vi "ControllerView.vi"() -> ()   [LabVIEW 2016]
uses:
  DataTypes/Topics/Parts/SummaryStates.ctl
  DataTypes/Topics/Parts/Timestamp.ctl
  Boot/Boot.lvclass
  UserEvents/UserEvents.lvclass/UserEvents.ctl
  DataTypes/General/ShutdownEvent.ctl
  Settings/Settings/Setting.lvclass
  UserEvents/UserEvents.lvclass
  DataTypes/General/M1M3SupportGeneral.lvlib
  DataTypes/Topics/M1M3SupportTopics.lvlib
panel:
  in  "Shutdown":bool
  out "SAL Time (ms)":i32=-123123
  in  "EditM1M3Settings":bool
  out "ModbusSubnetATxFrameCount":i32
  out "DeltaTimestamp":dbl format="%.6g"
  out "Timestamp":T1
  out "FPGATimestamp":dbl format="%.6g"
  in  "EditBaseSettings":bool
  out "SummaryStates":T2
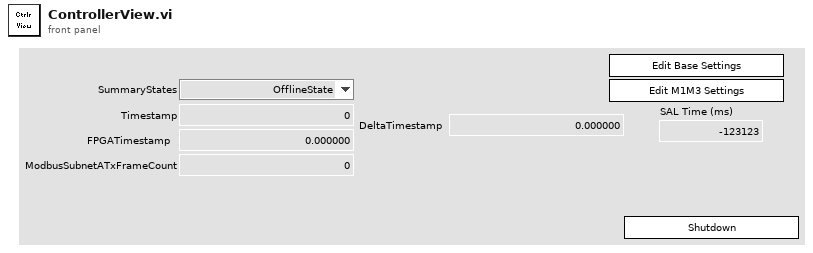
[diagram p1: front panel]
types:
  T1 = typedef "M1M3SupportTopics.lvlib/Timestamp.ctl" = dbl
  T2 = typedef "M1M3SupportTopics.lvlib/SummaryStates.ctl" = enum16{"OfflineState", "StandbyState", "DisabledState", "EnabledState", "FaultState"}
  T3 = enum32{"invalid app kind", "Development System", "Run Time System", "Student Edition", "Embedded LabVIEW", "Evaluation", "Custom"}
  T4 = typedef "M1M3SupportGeneral.lvlib/ShutdownEvent.ctl" = cluster{"Shutdown":bool}
  T5 = typedef "M1M3SupportTypes.lvlib/SummaryStates.ctl" = enum16{"OfflineState", "StandbyState", "DisabledState", "EnabledState", "FaultState"}
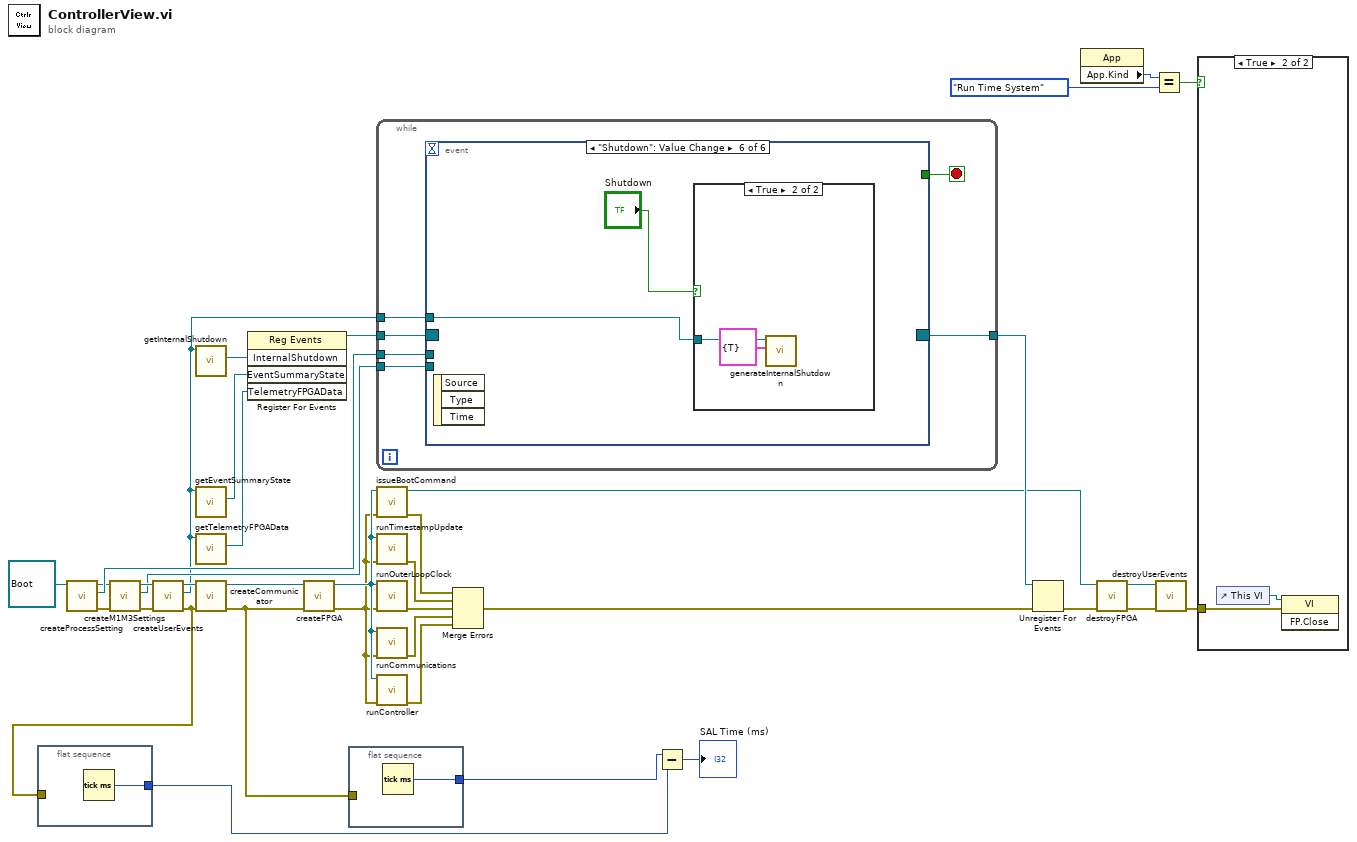
[diagram p0: block diagram]
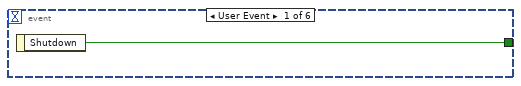
[diagram p3: hidden frame]
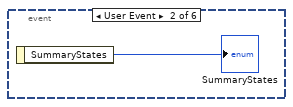
[diagram p4: hidden frame]
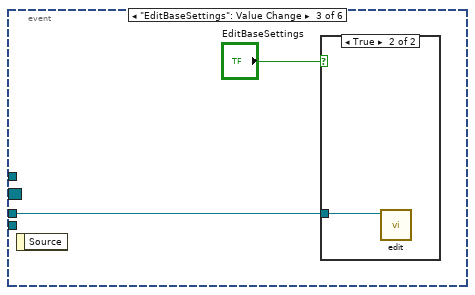
[diagram p5: hidden frame]
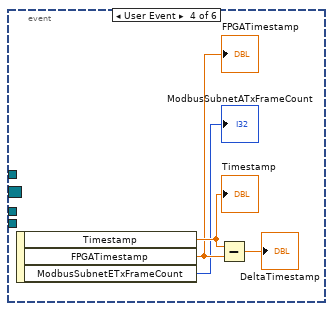
[diagram p7: hidden frame]
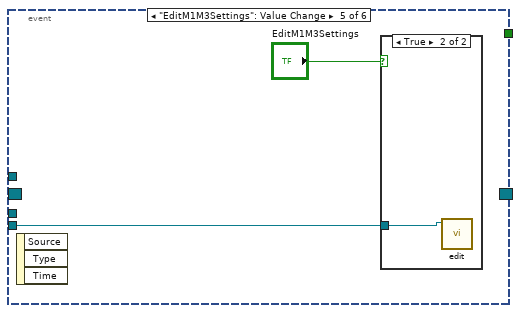
[diagram p8: hidden frame]
diagram:
  n1 = flat-sequence {
    tunnel: w6 -> [_]
    tunnel: [w37] -> w3
    frame #0 {
      n2 = Tick Count (ms)() -> (millisecond timer value=w37:u32)
    }
  }
  n3 = call "createProcessSetting.vi"("Boot in"=refnum<class "Boot.lvclass"> refnum ("Boot.lvclass")) -> ("error out"=w9:errorcluster, "ProcessSettings"=w23:refnum<class "Setting.lvclass">, "Boot out"=w11:refnum<class "Boot.lvclass">)  [unwired: 8 in]
  n4 = call "createM1M3Settings.vi"("error in (no error)"=w9, "Boot in"=w11) -> ("error out"=w8:errorcluster, "M1M3Settings"=w7:refnum<class "Setting.lvclass">, "Boot out"=w10:refnum<class "Boot.lvclass">)  [unwired: 7 in]
  n5 = call "createUserEvents.vi"("error in (no error)"=w8, "Boot in"=w10) -> ("error out"=w6:errorcluster, "UserEvents"=w1:refnum<class "UserEvents.lvclass">, "Boot out"=w14:refnum<class "Boot.lvclass">)  [unwired: 7 in]
  n6 = call "getInternalShutdown.vi"("UserEvents in"=w1) -> ("InternalShutdown"=w36:refnum<user-event>)  [unwired: 9 in, 1 out]
  n7 = call "getEventSummaryState.vi"("UserEvents in"=w1) -> ("EventSummaryState"=w35:refnum<user-event>)  [unwired: 9 in, 1 out]
  n8 = call "getTelemetryFPGAData.vi"("UserEvents in"=w1) -> ("TelemetryFPGAData"=w22:refnum<user-event>)  [unwired: 9 in, 1 out]
  n9 = call "createCommunicator.vi"("error in (no error)"=w6, "Boot in"=w14) -> ("error out"=w5:errorcluster, "Boot out"=w13:refnum<class "Boot.lvclass">)  [unwired: 7 in, 1 out]
  n10 = register-events(w36, w35, w22) -> (reference out=w34:refnum<event-registration>)  [unwired: 2 in, 1 out]
  n11 = call "createFPGA.vi"("error in (no error)"=w5, "Boot in"=w13) -> ("error out"=w20:errorcluster, "Boot out"=w21:refnum<class "Boot.lvclass">)  [unwired: 7 in, 1 out]
  n12 = flat-sequence {
    tunnel: w5 -> [_]
    tunnel: [w38] -> w4
    frame #0 {
      n13 = Tick Count (ms)() -> (millisecond timer value=w38:u32)
    }
  }
  n14 = while {
    tunnel: w34 -> [w44]
    tunnel: [w42] -> w33
    tunnel: w23 -> [w41]
    tunnel: w7 -> [w40]
    tunnel: w1 -> [w39]
    stop <- w43 stop-if-true
    n15 = event shown="[5] \"Shutdown\": Value Change" {
      selector: w44 -> [_ _ _ _ _ _]
      dyn-events: [_ _ _ _ _ _] -> w42
      timeout: _ -> [_ _ _ _ _ _]
      tunnel: [w45 _ _ _ _ _] -> w43
      tunnel: w41 -> [_ _ w47 _ _ _]
      tunnel: w40 -> [_ _ _ _ w54 _]
      tunnel: w39 -> [_ _ _ _ _ w57]
      event User Event {
        n16 = event-data() -> ("Shutdown"=w45:bool)  [unwired: 1 in]
      }
      event User Event {
        n17 = event-data() -> ("SummaryStates"=→"SummaryStates":T5)  [unwired: 1 in]
      }
      event "EditBaseSettings": Value Change {
        n18 = event-data() -> ()  [unwired: 1 in, 1 out]
        n19 = case shown="True" "EditBaseSettings" {
          tunnel: w47 -> [_ w49]
          frame False {
          }
          frame True {
            n20 = call-dynamic "edit.vi"("BaseSetting in"=w49) -> ()  [unwired: 8 in, 3 out]
          }
        }
      }
      event User Event {
        n21 = event-data() -> ("Timestamp"=w53:T1, "FPGATimestamp"=w52:dbl, "ModbusSubnetETxFrameCount"=→"ModbusSubnetATxFrameCount":u32)  [unwired: 1 in]
        "FPGATimestamp" <- w52
        "Timestamp" <- w53
        n22 = Subtract(x=w53, y=w52) -> (x-y=→"DeltaTimestamp":T1)
      }
      event "EditM1M3Settings": Value Change {
        n23 = event-data() -> ()  [unwired: 1 in, 3 out]
        n24 = case shown="True" "EditM1M3Settings" {
          tunnel: w54 -> [_ w56]
          frame False {
          }
          frame True {
            n25 = call-dynamic "edit.vi"("BaseSetting in"=w56) -> ()  [unwired: 8 in, 3 out]
          }
        }
      }
      event "Shutdown": Value Change {
        n26 = event-data() -> ()  [unwired: 1 in, 3 out]
        n27 = case shown="True" "Shutdown" {
          tunnel: w57 -> [_ w60]
          frame False {
          }
          frame True {
            n28 = call "generateInternalShutdown.vi"("ShutdownEvent"=T4 {"Shutdown"=TRUE}, "UserEvents in"=w60) -> ()  [unwired: 8 in, 2 out]
          }
        }
      }
    }
  }
  n29 = call "issueBootCommand.vi"("error in (no error)"=w20, "Boot in"=w21) -> ("error out"=w19:errorcluster, "Boot out"=w26:refnum<class "Boot.lvclass">)  [unwired: 8 in]
  n30 = call "runTimestampUpdate.vi"("error in (no error)"=w20, "Boot in"=w21) -> ("error out"=w18:errorcluster)  [unwired: 8 in, 1 out]
  n31 = call "runOuterLoopClock.vi"("error in (no error)"=w20, "Boot in"=w21) -> ("error out"=w17:errorcluster)  [unwired: 8 in, 1 out]
  n32 = call "runCommunications.vi"("error in (no error)"=w20, "Boot in"=w21) -> ("error out"=w16:errorcluster)  [unwired: 8 in, 1 out]
  n33 = call "runController.vi"("error in (no error)"=w20, "Boot in"=w21) -> ("error out"=w15:errorcluster)  [unwired: 8 in, 1 out]
  n34 = Merge Errors(w19, w18, w17, w16, w15) -> (w12:errorcluster)
  n35 = Subtract(x=w4, y=w3) -> (x-y=→"SAL Time (ms)":u32)
  n36 = Unregister For Events(event registration refnum=w33, error in=w12) -> (error out=w28:errorcluster)
  n37 = property class="App"() -> ("App.Kind"=w32:T3)  [unwired: 2 in, 2 out]
  n38 = call "destroyFPGA.vi"("error in (no error)"=w28, "Boot in"=w26) -> ("error out"=w27:errorcluster, "Boot out"=w25:refnum<class "Boot.lvclass">)  [unwired: 8 in]
  n39 = Equal?(x=w32, y=T3."Run Time System") -> (x = y?=w30:bool)
  n40 = call "destroyUserEvents.vi"("error in (no error)"=w27, "Boot in"=w25) -> ("error out"=w29:errorcluster)  [unwired: 8 in, 1 out]
  n41 = case shown="True" w30 {
    tunnel: w29 -> [_ w61]
    frame False {
    }
    frame True {
      n42 = control-ref of="This VI"() -> (w62:refnum<vi>)
      n43 = invoke class="VI" method="FP.Close"(reference=w62, error in=w61) -> ()  [unwired: 1 in, 3 out]
    }
  }
